vi "Scripting_CleanUpTermWire.vi"(8 "error in":errorcluster, 11 "TermIn":refnum<vi>) -> (0 "error out":errorcluster, 3 "TermOut":refnum<vi>)   [LabVIEW 2012]
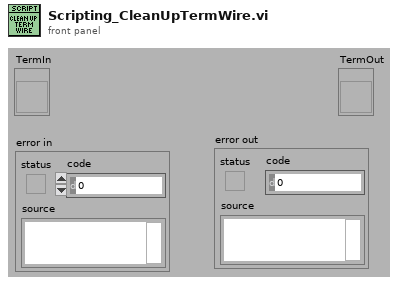
[diagram p1: front panel]
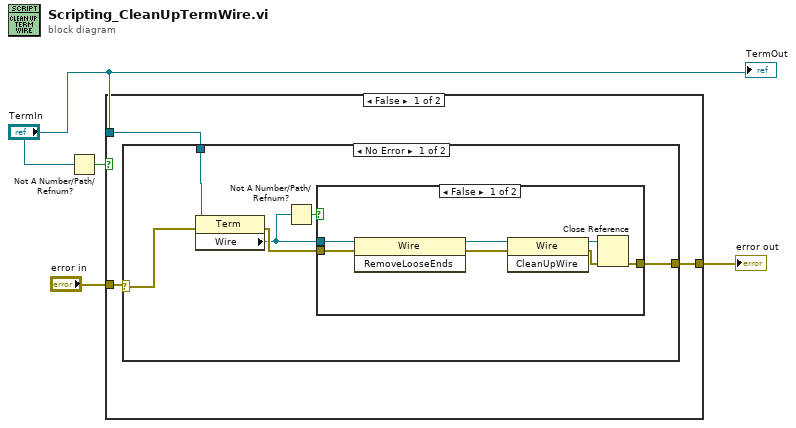
[diagram p0: block diagram]
diagram:
  n1 = Not A Number/Path/Refnum?(number/path/refnum="TermIn") -> (NaN/Path/Refnum?=w1:bool)
  n2 = case shown="False" w1 {
    tunnel: [w7 w23] -> w4
    tunnel: "error in" -> [w6 w23]
    tunnel: "TermIn" -> [w5 _]
    frame False {
      n3 = case shown="No Error" w6 {
        selector: w6 -> [w8 w22]
        tunnel: [w13 w22] -> w7
        tunnel: w5 -> [w9 _]
        frame No Error {
          n4 = property class="Term"(reference=w9, error in=w8) -> (error out=w12:errorcluster, "Wire"=w10:refnum<vi>)  [unwired: 1 out]
          n5 = Not A Number/Path/Refnum?(number/path/refnum=w10) -> (NaN/Path/Refnum?=w11:bool)
          n6 = case shown="False" w11 {
            tunnel: w10 -> [w17 _]
            tunnel: w12 -> [w16 w21]
            tunnel: [w18 w21] -> w13
            frame False {
              n7 = invoke class="Wire" method="RemoveLooseEnds"(reference=w17, error in=w16) -> (reference out=w14:refnum<vi>, error out=w15:errorcluster)  [unwired: 1 in, 1 out]
              n8 = invoke class="Wire" method="CleanUpWire"(reference=w14, error in=w15) -> (reference out=w20:refnum<vi>, error out=w19:errorcluster)  [unwired: 1 in, 1 out]
              n9 = Close Reference(reference=w20, error in (no error)=w19) -> (error out=w18:errorcluster)
            }
            frame True {
            }
          }
        }
        frame Error {
        }
      }
    }
    frame True {
    }
  }
  "error out" <- w4
  "TermOut" <- "TermIn"
